vi "test0627.vi"() -> ()   [LabVIEW 2017]
panel:
  in  "Impedance":u32(ring)=2 items=["1 MOhm"=1, "50 Ohm"=2, ""=0]
  in  "Range":u32(ring)=10 items=["20 mV"=1, "40 mV"=2, "50 mV"=3, "80 mV"=4, "100 mV"=5, "200 mV"=6, "400 mV"=7, "500 mV"=8, "800 mV"=9, "1 V"=10, "1.25 V"=33, "2 V"=11, "4 V"=12, "5 V"=13, "8 V"=14, "10 V"=15, "20 V"=16]
  in  "Coupling":u32(ring)=2 items=["AC"=1, "DC"=2]
  in  "Channel":u8(ring)=1 items=["A"=1, "B"=2, "C"=4, "D"=8]
  out "Handle 2":u32
  out "Return Code 2":u32
  out "error out 2":errorcluster
  in  "Decimation":u32
  in  "Edge":u32(ring) items=["Rising", "Falling"]
  in  "Sample Rate":u32(ring)=30 items=["1 kS/s"=1, "2 kS/s"=2, "5 kS/s"=4, "10 kS/s"=8, "20 kS/s"=10, "50 kS/s"=12, "100 kS/s"=14, "200 kS/s"=16, "500 kS/s"=18, "1 MS/s"=20, "2 MS/s"=24, "5 MS/s"=26, "10 MS/s"=28, "20 MS/s"=30, "25 MS/s"=33, "50 MS/s"=34, "100 MS/s"=36, "125 MS/s"=37, "160 MS/s"=38, "180 MS/s"=39, "250 MS/s"=43, "500 MS/s"=48, "800 MS/s"=50, "1000 MS/s"=53, "1200 MS/s"=55, "1500 MS/s"=58, "1800 MS/s"=61]
  in  "Source":u32(ring)=1 items=["Internal"=1, "Fast External"=2, "Medium External"=3, "Slow External"=4, "External AC"=5, "External DC"=6, "External 10MHz"=7]
  in  "System ID":i32
  in  "State":bool
  out "Return Code":u32
  in  "error in (no error)":errorcluster
  out "error out":errorcluster
  out "Handle":u32
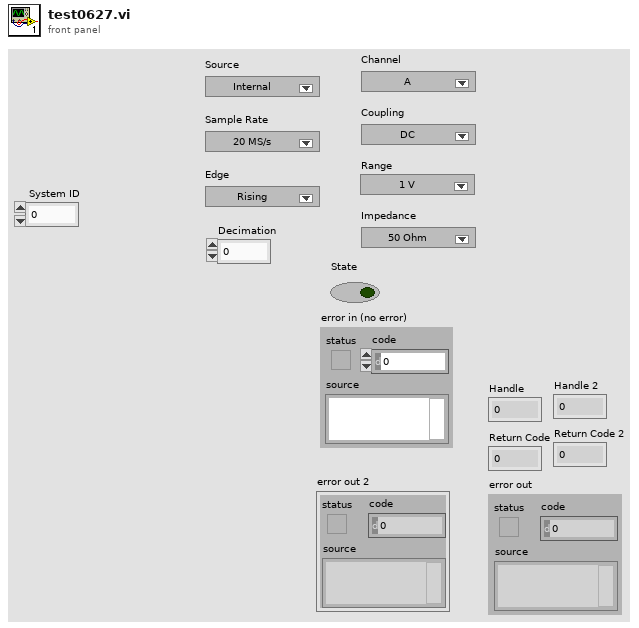
[diagram p1: front panel]
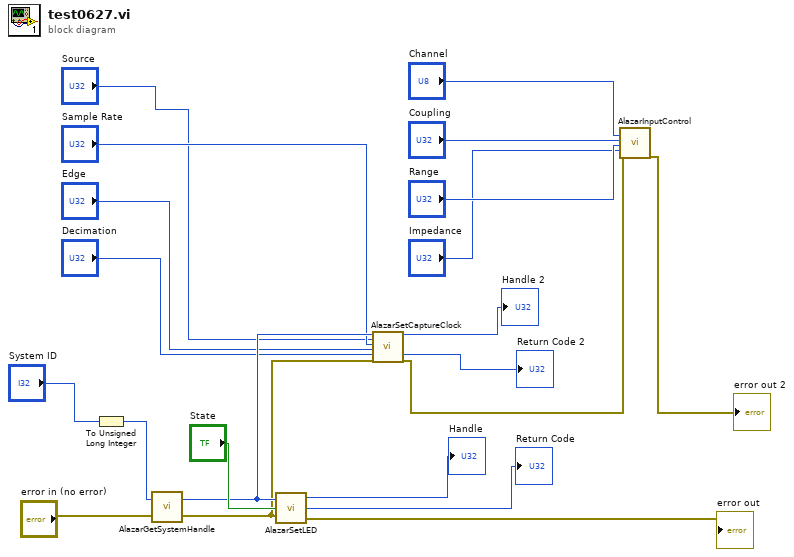
[diagram p0: block diagram]
diagram:
  n1 = To Unsigned Long Integer(number="System ID") -> (unsigned 32bit integer=w15:u32)
  n2 = call <vilib>:"AlazarGetSystemHandle.vi"("error in (no error)"="error in (no error)", "System ID"=w15) -> ("error out"=w3:errorcluster, "Handle"=w14:u32)
  n3 = call <vilib>:"AlazarSetLED.vi"("error in (no error)"=w3, "State"="State", "Handle"=w14) -> ("error out"=→"error out":errorcluster, "Return Code"=→"Return Code":u32, "Handle"=→"Handle":u32)
  n4 = call <vilib>:"AlazarSetCaptureClock.vi"("Handle"=w14, "Source"="Source", "Sample Rate"="Sample Rate", "Edge"="Edge", "Decimation"="Decimation", "error in (no error)"=w3) -> ("Handle"=→"Handle 2":u32, "Return Code"=→"Return Code 2":u32, "error out"=w2:errorcluster)  [unwired: 11 in]
  n5 = call <vilib>:"AlazarInputControl.vi"("Channel"="Channel", "Coupling"="Coupling", "Range"="Range", "Impedance"="Impedance", "error in (no error)"=w2) -> ("error out"=→"error out 2":errorcluster)  [unwired: 12 in, 2 out]
